vi "getAngle.vi"(0 "SPI Config In":T1) -> (1 "SPI Config Out":T1, 2 "Angle":fxp<+/-,32,16>, 3 "Transmit Error":bool)   [LabVIEW 2019]
uses:
  SPI/SPI Config.ctl
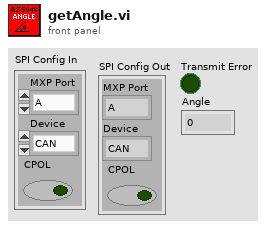
[diagram p1: front panel]
types:
  T1 = typedef "SPI Config.ctl" = cluster{"MXP Port":enum16{"A", "B"}, "Device":enum16{"CAN", "ENC", "IMU1", "IMU2"}, "CPOL":bool}
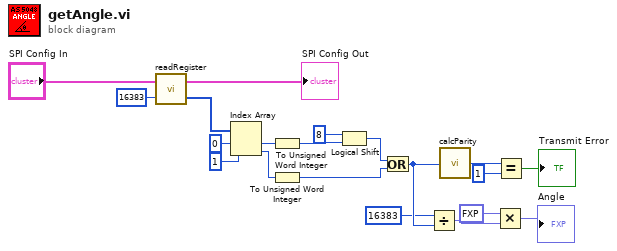
[diagram p0: block diagram]
diagram:
  n1 = call "readRegister.vi"("Register to Read"=u16 16383, "SPI Config In"="SPI Config In") -> ("Register Data Out"=w17:u8[], "SPI Config Out"=→"SPI Config Out":T1)
  n2 = Index Array(array=w17, index #1=0 ("index"), index #2=1 ("index")) -> (element #1=w14:u8, element #2=w11:u8)
  n3 = To Unsigned Word Integer(number=w14) -> (unsigned 16bit integer=w12:u16)
  n4 = To Unsigned Word Integer(number=w11) -> (unsigned 16bit integer=w9:u16)
  n5 = Logical Shift(y=i16 8, x=w12) -> (x << y=w10:u16)
  n6 = Or(x=w10, y=w9) -> (x .or. y?=w5:u16)
  n7 = Divide(x=u16 16383, y=w5) -> (x/y=w3:fxp<+/-,32,16>)
  n8 = call "calcParity.vi"("Number"=w5) -> ("Parity"=w8:u16)
  n9 = Multiply(x=fxp<+/-,32,16> 360.0, y=w3) -> (x*y=→"Angle":fxp<+/-,32,16>)
  n10 = Equal?(x=w8, y=u16 1) -> (x = y?=→"Transmit Error":bool)
